vi "VIP.vi"() -> ()   [LabVIEW 2017, in "Examples.lvlib"]
uses:
  Examples.lvlib
panel:
  out "Numeric":i32
  in  "stop":bool
  out "RealPower Waveform Chart":sgl(graph)
  out "F401130":sgl
  out "Current Waveform Chart":sgl(graph)
  out "F401122 Current":sgl
  out "Voltage Waveform Chart":sgl(graph)
  out "F401007 Voltage":sgl
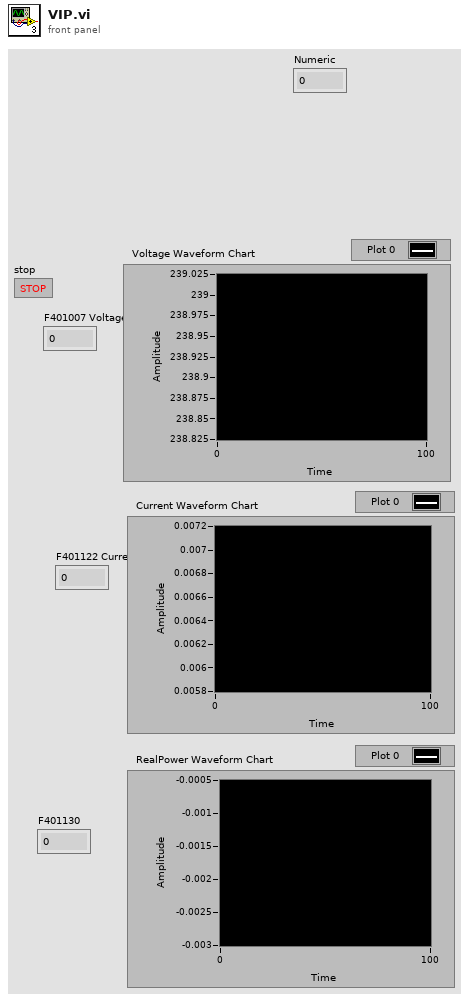
[diagram p1: front panel]
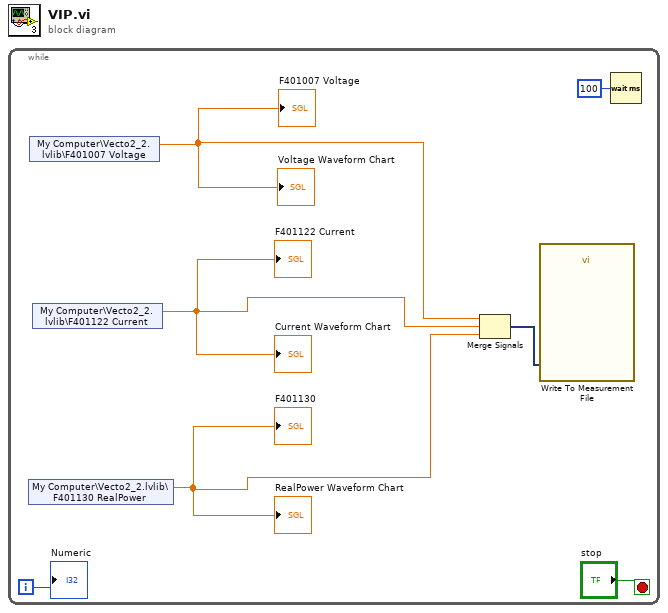
[diagram p0: block diagram]
diagram:
  n1 = while {
    i -> [w1]
    stop <- "stop" stop-if-true
    n2 = shared-variable "My Computer\\Vecto2_2.lvlib\\F401130 RealPower"() -> (w3:sgl)  [unwired: 1 in, 1 out]
    "F401130" <- w3
    "RealPower Waveform Chart" <- w3
    n3 = shared-variable "My Computer\\Vecto2_2.lvlib\\F401007 Voltage"() -> (w5:sgl)  [unwired: 1 in, 1 out]
    "F401007 Voltage" <- w5
    "Voltage Waveform Chart" <- w5
    n4 = shared-variable "My Computer\\Vecto2_2.lvlib\\F401122 Current"() -> (w4:sgl)  [unwired: 1 in, 1 out]
    "F401122 Current" <- w4
    "Current Waveform Chart" <- w4
    n5 = Merge Signals(w5, w4, w3) -> (w2:dynamicdata)
    n6 = call "Write To Measurement File"("Signals"=w2) -> ()  [unwired: 16 in, 3 out]
    n7 = Wait (ms)(milliseconds to wait=u32 100) -> ()  [unwired: 1 out]
    "Numeric" <- w1
  }
